vi "Refactor Parent Class Dependency.vi"(8 "error in (no error)":errorcluster, 10 "rename data":T1, 11 "project classes in":refnum<vi>[](array[refnum])) -> (0 "error out":errorcluster, 2 "refactored classes":path[](array[path]), 3 "project classes out":refnum<vi>[](array[refnum]))   [LabVIEW 2021, in "MeasurementService Editor.lvlib"]
uses:
  MeasurementService Editor.lvlib
  Rename Refactor Data.ctl
  Rename Refactor Mapping Info.ctl
  Rename String Mapping.ctl
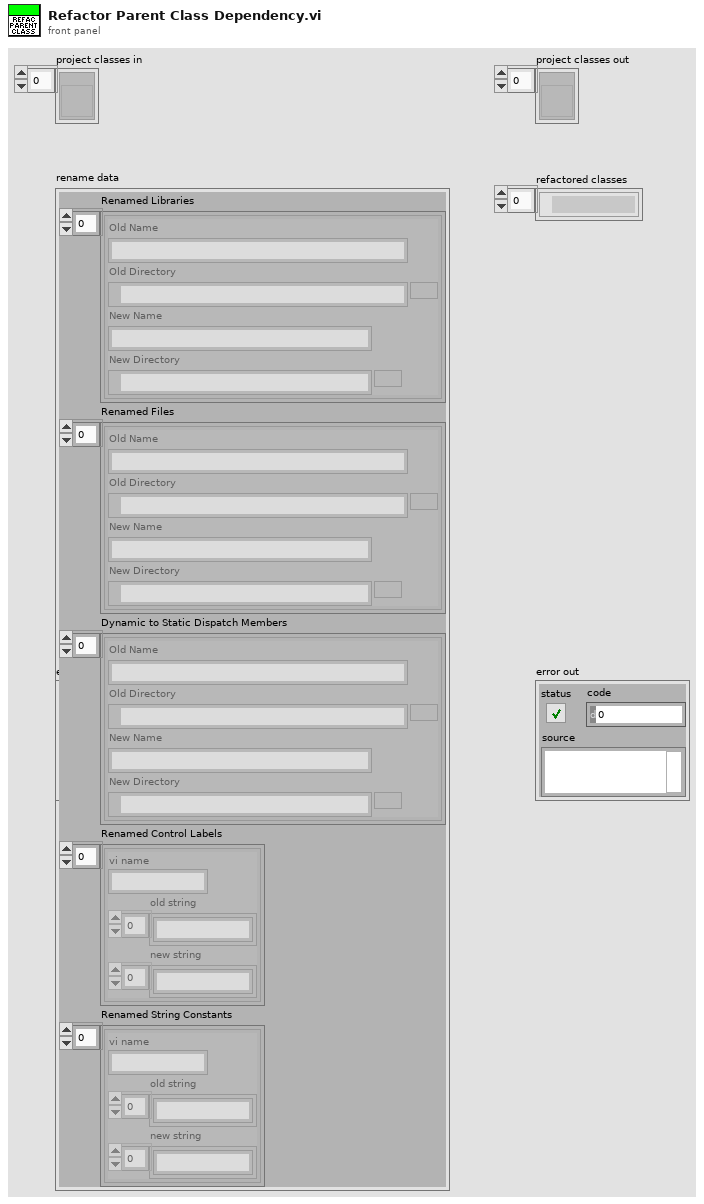
[diagram p1: front panel]
types:
  T1 = typedef "MeasurementService Editor.lvlib/Rename Refactor Data.ctl" = cluster{"Renamed Libraries":T2[], "Renamed Files":T2[], "Dynamic to Static Dispatch Members":T2[], "Renamed Control Labels":T3[], "Renamed String Constants":T3[]}
  T2 = typedef "MeasurementService Editor.lvlib/Rename Refactor Mapping Info.ctl" = cluster{"Old Name":string, "Old Directory":path, "New Name":string, "New Directory":path}
  T3 = typedef "MeasurementService Editor.lvlib/Rename String Mapping.ctl" = cluster{"vi name":string, "old string":string[], "new string":string[]}
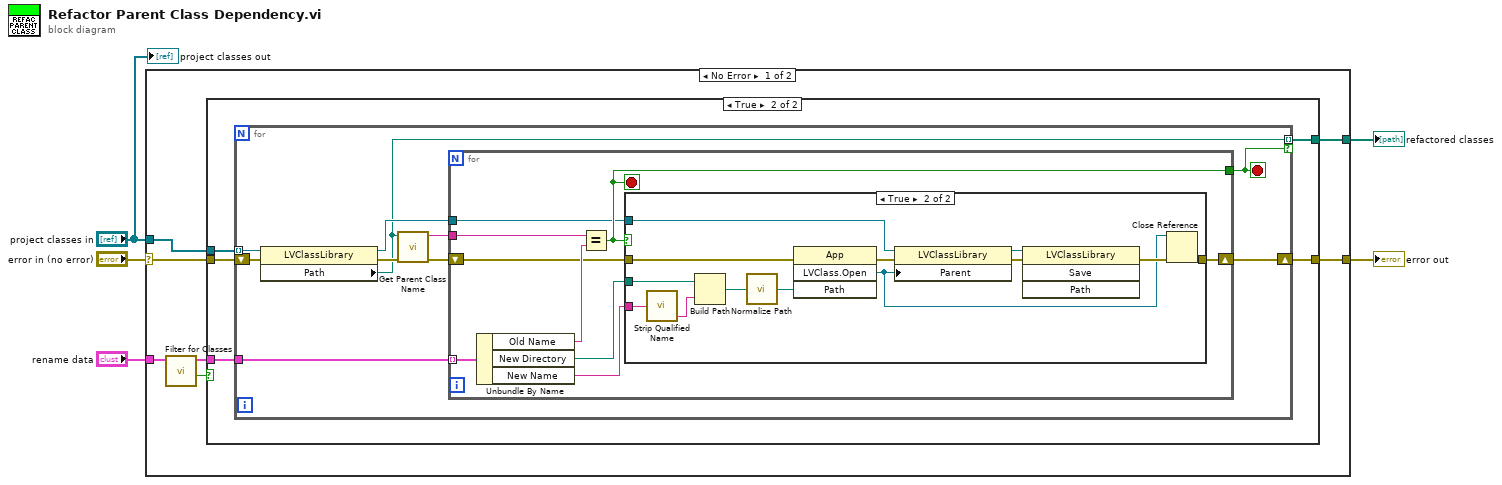
[diagram p0: block diagram]
diagram:
  n1 = case shown="No Error" "error in (no error)" {
    selector: "error in (no error)" -> [w11 w52]
    tunnel: [w12 w52] -> w5
    tunnel: [w10 _] -> w3
    tunnel: "project classes in" -> [w9 _]
    tunnel: "rename data" -> [w6 _]
    frame No Error {
      n2 = call "Filter for Classes.vi"("rename data"=w6) -> ("found classes?"=w7:bool, "renamed classes"=w8:T2[])  [unwired: 9 in]
      n3 = case shown="True" w7 {
        tunnel: [w13 w18] -> w12
        tunnel: w11 -> [w13 w17]
        tunnel: [_ w16] -> w10
        tunnel: w9 -> [_ w15]
        tunnel: w8 -> [_ w14]
        frame False {
        }
        frame True {
          n4 = for {
            tunnel: w15 -> [w19] mode=indexing
            tunnel: w14 -> [w27]
            shift-right: [w23] -> w18
            shift-left: w17 -> [w20]
            tunnel: [w22] -> w16 mode=indexing if=w21
            stop <- w21 stop-if-true
            n5 = property class="LVClassLibrary"(reference=w19, error in=w20) -> (reference out=w24:refnum<vi>, error out=w28:errorcluster, "Path"=w22:path)
            n6 = call "Get Parent Class Name.vi"("error in (no error)"=w28, "lvclass path"=w22) -> ("error out"=w25:errorcluster, "parent class name"=w26:string)  [unwired: 8 in]
            n7 = for {
              tunnel: w27 -> [w37] mode=indexing
              tunnel: w26 -> [w35]
              tunnel: [w34] -> w21
              shift-right: [w29] -> w23
              shift-left: w25 -> [w33]
              tunnel: w24 -> [w30]
              stop <- w34 stop-if-true
              n8 = Unbundle By Name(w37) -> ("Old Name"=w36:string, "New Directory"=w32:path, "New Name"=w31:string)
              n9 = Equal?(x=w35, y=w36) -> (x = y?=w34:bool)
              n10 = case shown="True" w34 {
                tunnel: w33 -> [w38 w50]
                tunnel: w32 -> [_ w51]
                tunnel: w31 -> [_ w42]
                tunnel: w30 -> [_ w49]
                tunnel: [w38 w44] -> w29
                frame False {
                }
                frame True {
                  n11 = call "Strip Qualified Name.vi"("name"=w42) -> ("last name"=w41:string)  [unwired: 5 in, 1 out]
                  n12 = Build Path(base path=w51, name or relative path=w41) -> (appended path=w40:path)
                  n13 = call "Normalize Path.vi"("path"=w40) -> ("normalized path"=w39:path)
                  n14 = invoke class="App" method="LVClass.Open"(error in=w50, "Path"=w39) -> (error out=w48:errorcluster, "LVClass.Open"=w43:refnum<vi>)  [unwired: 2 in, 2 out]
                  n15 = property class="LVClassLibrary"(reference=w49, error in=w48, "Parent"=w43) -> (reference out=w47:refnum<vi>, error out=w46:errorcluster)
                  n16 = invoke class="LVClassLibrary" method="Save"(reference=w47, error in=w46) -> (error out=w45:errorcluster)  [unwired: 2 in, 3 out]
                  n17 = Close Reference(reference=w43, error in (no error)=w45) -> (error out=w44:errorcluster)
                }
              }
            }
          }
        }
      }
    }
    frame Error {
    }
  }
  "error out" <- w5
  "refactored classes" <- w3
  "project classes out" <- "project classes in"
